vi "magnetTest.vi"() -> ()   [LabVIEW 2020]
panel:
  out "Steps":dbl
  in  "Max Voltage":dbl
  in  "Wait Time":i32(knob) scale=0.0..5000.0
  in  "Loops":i32
  out "Loop\n Number":dbl
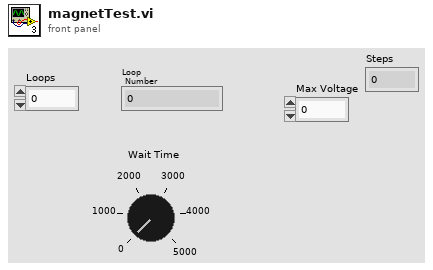
[diagram p1: front panel]
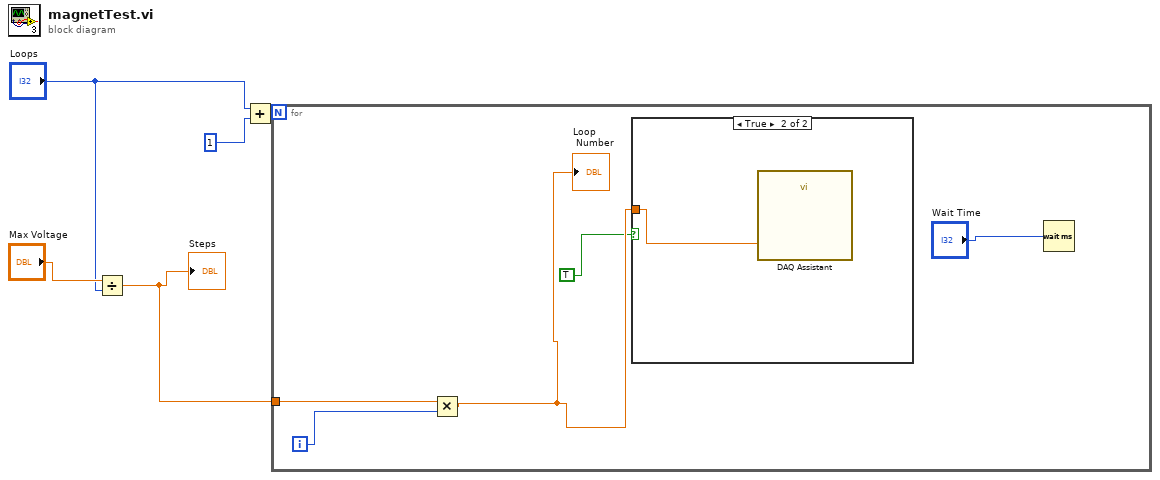
[diagram p0: block diagram]
diagram:
  n1 = Divide(x="Max Voltage", y="Loops") -> (x/y=w1:dbl)
  "Steps" <- w1
  n2 = Add(x="Loops", y=1) -> (x+y=w5:i32)
  n3 = for {
    N: w5 -> [_]
    tunnel: w1 -> [w7]
    i -> [w8]
    n4 = Multiply(x=w7, y=w8) -> (x*y=w9:dbl)
    "Loop\n Number" <- w9
    n5 = case shown="True" TRUE {
      tunnel: w9 -> [_ w11]
      frame False {
      }
      frame True {
        n6 = call "DAQ Assistant"("data"=w11) -> ()  [unwired: 17 in, 2 out]
      }
    }
    n7 = Wait (ms)(milliseconds to wait="Wait Time") -> ()  [unwired: 1 out]
  }
